vi "Prepare SQL Statements_BW.vi"(7 "action":enum16{"Init", "Read", "Finalise"}(ring), 8 "error in (no error)":errorcluster, 11 "SQLite Connection in":refnum<class "Connection.lvclass">) -> (0 "error out":errorcluster, 1 "Readings":refnum<class "SQL Statement.lvclass">, 2 "Events":refnum<class "SQL Statement.lvclass">, 3 "SQLite Connection out":refnum<class "Connection.lvclass">, 4 "REadingVal":refnum<class "SQL Statement.lvclass">)   [LabVIEW 2017]
doc: "Adds a new album to the database."
uses:
  <vilib>/drjdpowell/SQLite Library/SQL Connection/Connection.lvclass
  SQL Statements.ctl
  <vilib>/drjdpowell/SQLite Library/SQL Statement/SQL Statement.lvclass
  Common64/Database/SQ Lite/SQ Lite Cluster Action.ctl
  <vilib>/drjdpowell/SQLite Library/SQL Statement/SQL Statement.lvclass/SQL Statement.ctl
  Beltwatch/BeltWatch 4-2-2-5/Database/Beltwatch SQLite.lvlib
panel:
  out "Time":u32
  out "BW SQL Statements":T1
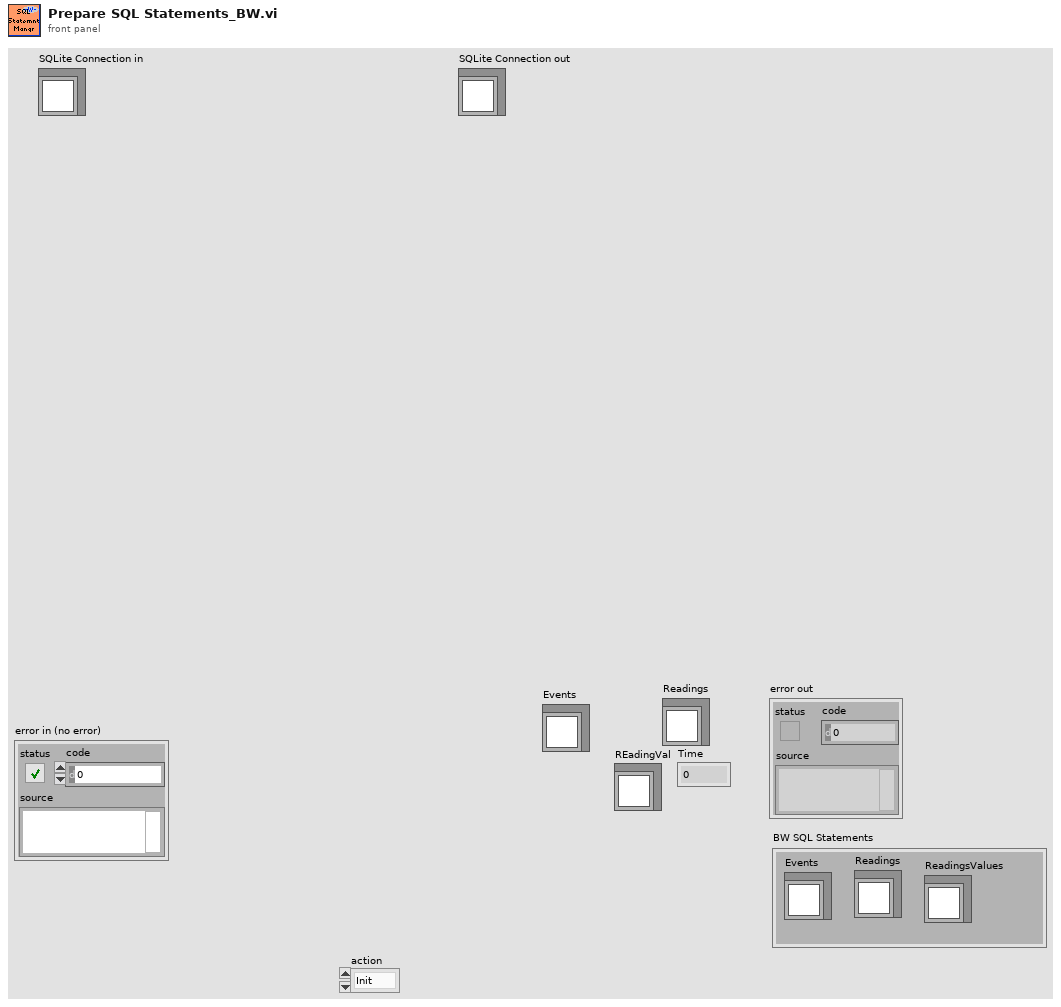
[diagram p1: front panel]
types:
  T1 = typedef "SQL Statements.ctl" = cluster{"Events":refnum<class "SQL Statement.lvclass">, "Readings":refnum<class "SQL Statement.lvclass">, "ReadingsValues":refnum<class "SQL Statement.lvclass">}
  T2 = typedef "Beltwatch SQLite.lvlib/SQ Lite Cluster Action.ctl" = cluster{"Include":bool, "Name":string, "SQLite3 type":enum32{"undefined type (0)", "SQLITE_INTEGER", "SQLITE_FLOAT", "SQLITE3_TEXT", "SQLITE_BLOB", "SQLITE_NULL", "undefined type"}}
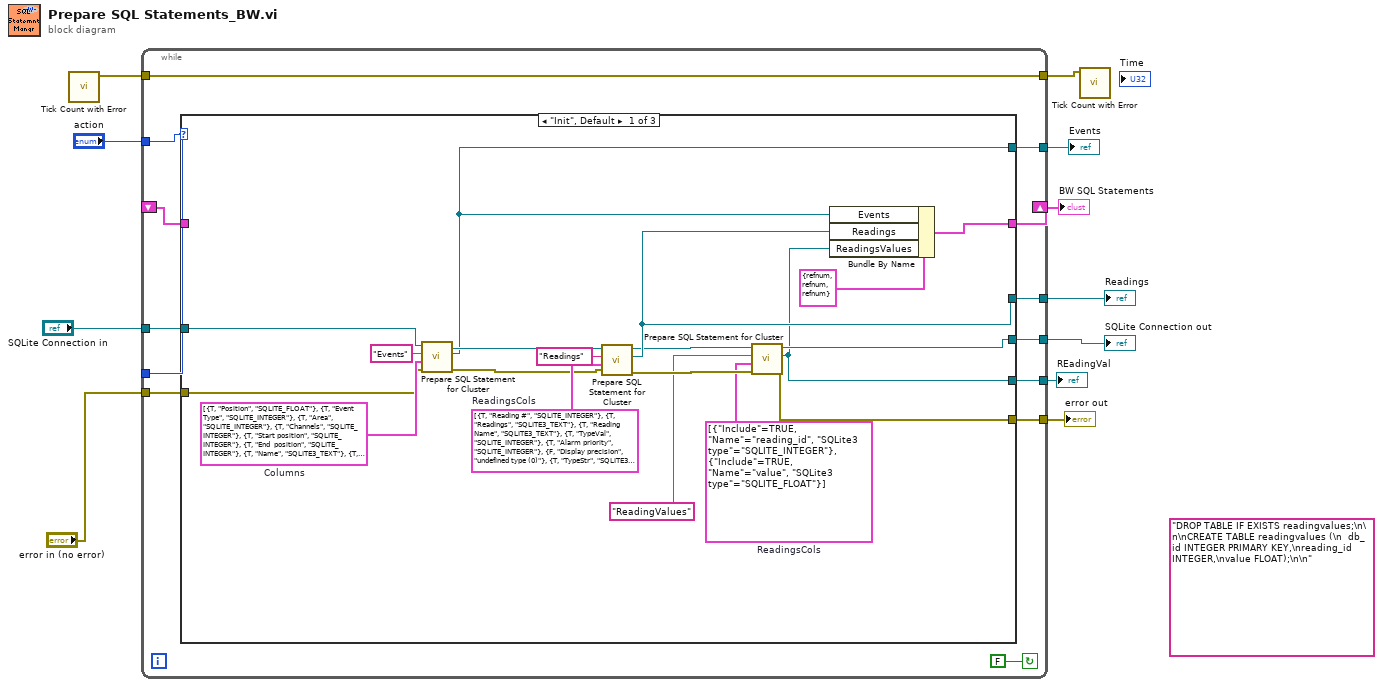
[diagram p0: block diagram]
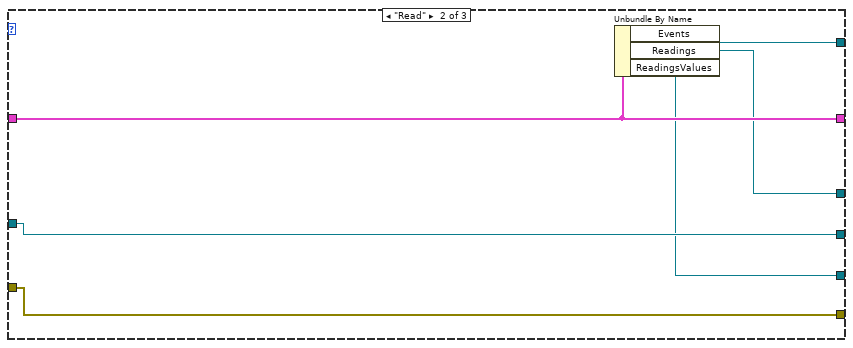
[diagram p2: hidden frame]
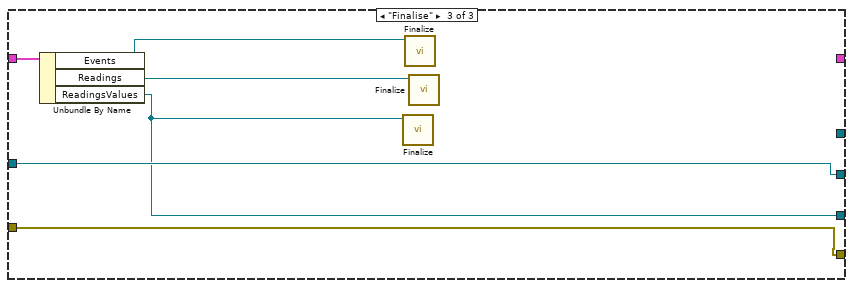
[diagram p3: hidden frame]
diagram:
  (unwired) "DROP TABLE IF EXISTS readingvalues;\n\n\nCREATE TABLE readingvalues (\n  db_id INTEGER PRIMARY KEY,\nreading_id INTEGER,\nvalue FLOAT);\n\n" ("Pre String")
  n1 = call "Tick Count with Error.vi"() -> ("error out"=w2:errorcluster)  [unwired: 9 in, 2 out]
  n2 = while {
    tunnel: [w14] -> _
    shift-right: [w23] -> w11
    shift-left: _ -> [w21]
    tunnel: [w20] -> w10
    tunnel: [w19] -> w9
    tunnel: "error in (no error)" -> [w18]
    tunnel: [w17] -> w7
    tunnel: [w16] -> w6
    tunnel: "SQLite Connection in" -> [w15]
    tunnel: "action" -> [w14]
    tunnel: [w13] -> w3
    tunnel: w2 -> [w12]
    tunnel: [w12] -> w1
    stop <- FALSE continue-if-true
    n3 = case shown="\"Init\", Default" w14 {
      tunnel: [w37 w48 _] -> w23
      tunnel: w21 -> [_ w48 w54]
      tunnel: [w36 w47 _] -> w20
      tunnel: [w35 w46 _] -> w19
      tunnel: w18 -> [w34 w45 w50]
      tunnel: [w25 w45 w50] -> w17
      tunnel: [w26 w44 w51] -> w16
      tunnel: w15 -> [w31 w44 w51]
      tunnel: [w24 w43 w49] -> w13
      frame "Init", Default {
        w27 = T2[] [{"Include"=TRUE, "Name"="reading_id", "SQLite3 type"=enum."SQLITE_INTEGER"}, {"Include"=TRUE, "Name"="value", "SQLite3 type"=enum."SQLITE_FLOAT"}]  # ReadingsCols
        w40 = T2[] [{"Include"=TRUE, "Name"="Reading #", "SQLite3 type"=enum."SQLITE_INTEGER"}, {"Include"=TRUE, "Name"="Readings", "SQLite3 type"=enum."SQLITE3_TEXT"}, {"Include"=TRUE, "Name"="Reading Name", "SQLite3 type"=enum."SQLITE3_TEXT"}, {"Include"=TRUE, "Name"="TypeVal", "SQLite3 type"=enum."SQLITE_INTEGER"}, {"Include"=TRUE, "Name"="Alarm priority", "SQLite3 type"=enum."SQLITE_INTEGER"}, {"Include"=FALSE, "Name"="Display precision", "SQLite3 type"=enum."undefined type (0)"}, {"Include"=TRUE, "Name"="TypeStr", "SQLite3 type"=enum."SQLITE3_TEXT"}, {"Include"=TRUE, "Name"="AlarmPriorityStr", "SQLite3 type"=enum."SQLITE3_TEXT"}]  # ReadingsCols
        w42 = T2[] [{"Include"=TRUE, "Name"="Position", "SQLite3 type"=enum."SQLITE_FLOAT"}, {"Include"=TRUE, "Name"="Event Type", "SQLite3 type"=enum."SQLITE_INTEGER"}, {"Include"=TRUE, "Name"="Area", "SQLite3 type"=enum."SQLITE_INTEGER"}, {"Include"=TRUE, "Name"="Channels", "SQLite3 type"=enum."SQLITE_INTEGER"}, {"Include"=TRUE, "Name"="Start position", "SQLite3 type"=enum."SQLITE_INTEGER"}, {"Include"=TRUE, "Name"="End  position", "SQLite3 type"=enum."SQLITE_INTEGER"}, {"Include"=TRUE, "Name"="Name", "SQLite3 type"=enum."SQLITE3_TEXT"}, {"Include"=TRUE, "Name"="Offset", "SQLite3 type"=enum."SQLITE_INTEGER"}, {"Include"=TRUE, "Name"="Length", "SQLite3 type"=enum."SQLITE_INTEGER"}, {"Include"=TRUE, "Name"="Action marker", "SQLite3 type"=enum."SQLITE3_TEXT"}, {"Include"=TRUE, "Name"="Event", "SQLite3 type"=enum."SQLITE_INTEGER"}, {"Include"=TRUE, "Name"="# Defects", "SQLite3 type"=enum."SQLITE_INTEGER"}, {"Include"=TRUE, "Name"="jpg Image", "SQLite3 type"=enum."SQLITE3_TEXT"}, {"Include"=TRUE, "Name"="chan maxs", "SQLite3 type"=enum."SQLITE_INTEGER"}, {"Include"=TRUE, "Name"="chan mins", "SQLite3 type"=enum."SQLITE_INTEGER"}, {"Include"=TRUE, "Name"="TimeStamp", "SQLite3 type"=enum."SQLITE_INTEGER"}, {"Include"=TRUE, "Name"="Readings", "SQLite3 type"=enum."SQLITE3_TEXT"}, {"Include"=TRUE, "Name"="ID", "SQLite3 type"=enum."SQLITE_INTEGER"}, {"Include"=TRUE, "Name"="New", "SQLite3 type"=enum."SQLITE_INTEGER"}, {"Include"=TRUE, "Name"="Hires Track", "SQLite3 type"=enum."SQLITE_INTEGER"}, {"Include"=TRUE, "Name"="2D overlay", "SQLite3 type"=enum."SQLITE_INTEGER"}, {"Include"=TRUE, "Name"="update", "SQLite3 type"=enum."SQLITE_INTEGER"}, {"Include"=TRUE, "Name"="Field #", "SQLite3 type"=enum."SQLITE_INTEGER"}, {"Include"=TRUE, "Name"="Events Class", "SQLite3 type"=enum."SQLITE_INTEGER"}, {"Include"=TRUE, "Name"="Sync", "SQLite3 type"=enum."SQLITE_INTEGER"}, {"Include"=TRUE, "Name"="Insert Offset", "SQLite3 type"=enum."SQLITE_INTEGER"}, {"Include"=TRUE, "Name"="Next trend", "SQLite3 type"=enum."SQLITE_INTEGER"}, {"Include"=TRUE, "Name"="Speed", "SQLite3 type"=enum."SQLITE_INTEGER"}]  # Columns
        n4 = call "Prepare SQL Statement for Cluster.vi"("error in (no error)"=w34, "Columns"=w42, "Table"="Events", "SQLite Connection in"=w31) -> ("error out"=w33:errorcluster, "SQL Statement"=w36:refnum<class "SQL Statement.lvclass">, "SQLite Connection out"=w41:refnum<class "Connection.lvclass">)  [unwired: 4 in, 1 out]
        n5 = call "Prepare SQL Statement for Cluster.vi"("error in (no error)"=w33, "Columns"=w40, "Table"="Readings", "SQLite Connection in"=w41) -> ("error out"=w29:errorcluster, "SQL Statement"=w35:refnum<class "SQL Statement.lvclass">, "SQLite Connection out"=w30:refnum<class "Connection.lvclass">)  [unwired: 4 in, 1 out]
        n6 = call "Prepare SQL Statement for Cluster.vi"("error in (no error)"=w29, "Columns"=w27, "Table"="ReadingValues", "SQLite Connection in"=w30) -> ("error out"=w25:errorcluster, "SQL Statement"=w24:refnum<class "SQL Statement.lvclass">, "SQLite Connection out"=w26:refnum<class "Connection.lvclass">)  [unwired: 4 in, 1 out]
        n7 = Bundle By Name(cluster=T1 {"Events"=refnum, "Readings"=refnum, "ReadingsValues"=refnum} ("BW SQL Statements"), "Events"=w36, "Readings"=w35, "ReadingsValues"=w24) -> (w37:T1)
      }
      frame "Read" {
        n8 = Unbundle By Name(w48) -> ("Events"=w47:refnum<class "SQL Statement.lvclass">, "Readings"=w46:refnum<class "SQL Statement.lvclass">, "ReadingsValues"=w43:refnum<class "SQL Statement.lvclass">)
      }
      frame "Finalise" {
        n9 = Unbundle By Name(w54) -> ("Events"=w53:refnum<class "SQL Statement.lvclass">, "Readings"=w52:refnum<class "SQL Statement.lvclass">, "ReadingsValues"=w49:refnum<class "SQL Statement.lvclass">)
        n10 = call <vilib>:"Finalize.vi"("SQL Statement in"=w49) -> ()  [unwired: 10 in, 1 out]
        n11 = call <vilib>:"Finalize.vi"("SQL Statement in"=w53) -> ()  [unwired: 10 in, 1 out]
        n12 = call <vilib>:"Finalize.vi"("SQL Statement in"=w52) -> ()  [unwired: 10 in, 1 out]
      }
    }
  }
  "SQLite Connection out" <- w6
  "BW SQL Statements" <- w11
  "Events" <- w10
  "Readings" <- w9
  "error out" <- w7
  "REadingVal" <- w3
  n13 = call "Tick Count with Error.vi"("error in (no error)"=w1) -> ()  [unwired: 8 in, 3 out]
